vi "2 Waypoint Monitor.vi"() -> ()   [LabVIEW 2011]
doc: "TODO: important As of 10/27 this VI only works for the Drive option\n\nWaypoint Monitor takes two things from the global variable - the list of waypoints and\nthe position of the robot at the time.\n\nIt compares the current position to the position of the current waypoint, and if that distance\nis less than the required accuracy the current waypoint value is incremented"
uses:
  0x2-OCU-Think Comm/0x2 Typedefs/waypointTypes.ctl
  2 Classes/Waypoint/Waypoint.lvclass
  2 Globals/2 Global.vi
panel:
  out "Target Distance/Time":dbl
  out "Distance to waypoint":dbl
  # "Waypoint Monitor takes two things from the global variable - the list of waypoints and\nthe position of the robot at the time.\n\nIt compares the current position to the position of the current waypoint, and if that distance\nis less than the required accuracy the current waypoint value is incremented\n\nTODO - Is there a way to only write the Current Waypoint?\nHow do you test something like this that is linked to the global?"
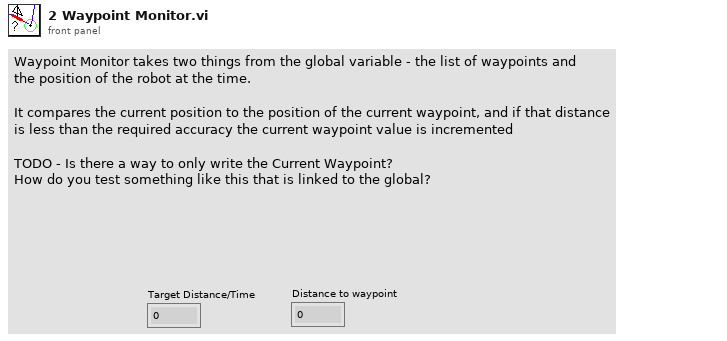
[diagram p1: front panel]
types:
  T1 = typedef "waypointTypes.ctl" = enum16{"Drive", "Round Port", "Round Starboard", "Stay"}
  T2 = typedef "Current Waypoint.ctl" = i32
  T3 = typedef "Waypoints List.ctl" = refnum<class "Waypoint.lvclass">[]
  T4 = typedef "UTM Location.ctl" = cluster{"UTM Zone":dbl, "Hemisphere":enum16{"North", "South"}, "East":dbl, "North":dbl}
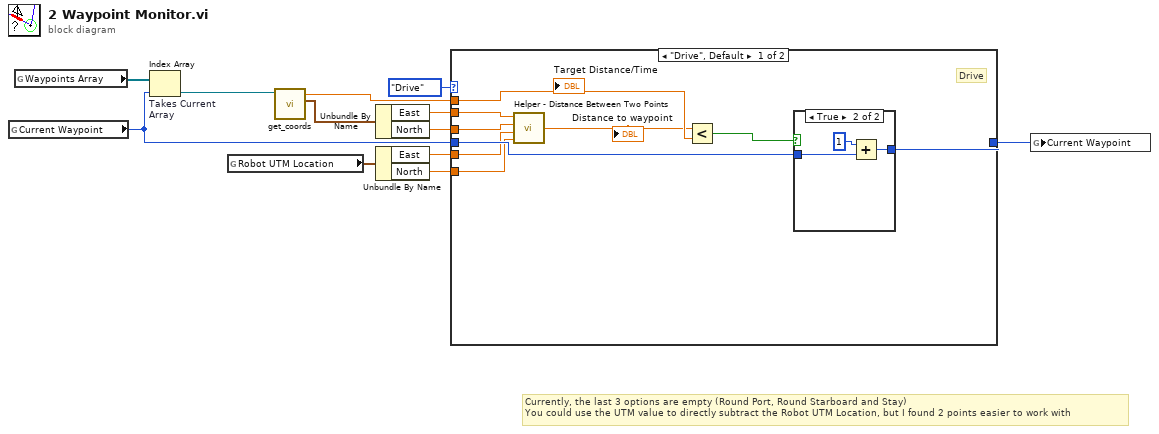
[diagram p0: block diagram]
diagram:
  # "Currently, the last 3 options are empty (Round Port, Round Starboard and Stay)\nYou could use the UTM value to directly subtract the Robot UTM Location, but I found 2 points easier to work with"
  n1 = global read "2 Global.vi" "Current Waypoint"() -> (w7:T2)
  n2 = global read "2 Global.vi" "Waypoints Array"() -> (w5:T3)
  n3 = Index Array "Takes Current\nArray"(array=w5, index=w7) -> (element=w1:refnum<class "Waypoint.lvclass">)
  n4 = global read "2 Global.vi" "Robot UTM Location"() -> (w12:T4)
  n5 = call-dynamic "get_coords.vi"("Waypoint in"=w1) -> ("Tolerance (meters?)"=w3:dbl, "Coords"=w2:T4)  [unwired: 7 in, 2 out]
  n6 = Unbundle By Name(w2) -> ("East"=w9:dbl, "North"=w8:dbl)
  n7 = Unbundle By Name(w12) -> ("East"=w11:dbl, "North"=w10:dbl)
  n8 = case shown="\"Drive\", Default" waypointTypes."Drive" ("Point Type") {
    tunnel: w3 -> [w21 _]
    tunnel: [w18 w26] -> w6
    tunnel: w7 -> [w19 w26]
    tunnel: w11 -> [w14 _]
    tunnel: w10 -> [w13 _]
    tunnel: w9 -> [w16 _]
    tunnel: w8 -> [w15 _]
    frame "Drive", Default {
      # "Drive"
      n9 = call "Helper - Distance Between Two Points.vi"("y 2"=w13, "x 2"=w14, "y"=w15, "x"=w16) -> ("Numeric"=w17:dbl)
      "Distance to waypoint" <- w17
      n10 = Less?(x=w17, y=w21) -> (x < y?=w20:bool)
      n11 = case shown="True" w20 {
        tunnel: w19 -> [w22 w25]
        tunnel: [w22 w23] -> w18
        frame False {
        }
        frame True {
          n12 = Add(x=1, y=w25) -> (x+y=w23:T2)
        }
      }
      "Target Distance/Time" <- w21
    }
    frame "Stay" {
      # "Stay"
    }
  }
  n13 = global write "2 Global.vi" "Current Waypoint"(w6) -> ()
